vi "dataUnwrapperToplevel.vi"(0 "dataIn":u32[](array[numeric])=[814743552, 16777221, 16777621, 16778021, 814745600, 16777221, 16777621, 16778021, 814747648, 16777221, 16777621, 16778021, 814749696, 16777221, 16777621, 16778021, 814751744, 16777221, 16777621, 16778021, 814753792, 16777221, 16777621, 16778021, 0] format="%032b", 2 "nOfSteps":i32=6, 4 "nOfScans":i32=1) -> (10 "DataUntouchedOut":u32[](array[numeric]), 14 "VoltArray":u32[](array[numeric]) format="%032b", 16 "CounterArray":u32[][][](array[numeric]), 18 "TRSArray":u32[][][](array[numeric]))   [LabVIEW 2014]
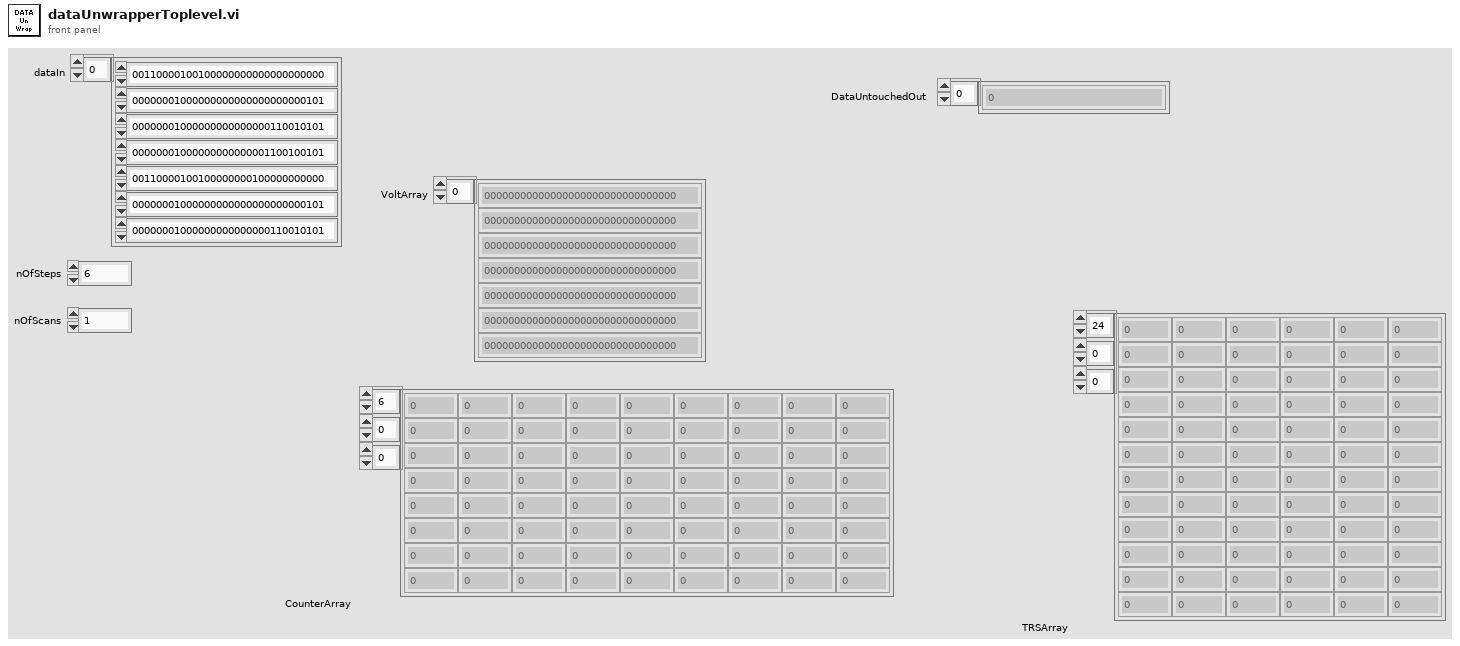
[diagram p1: front panel]
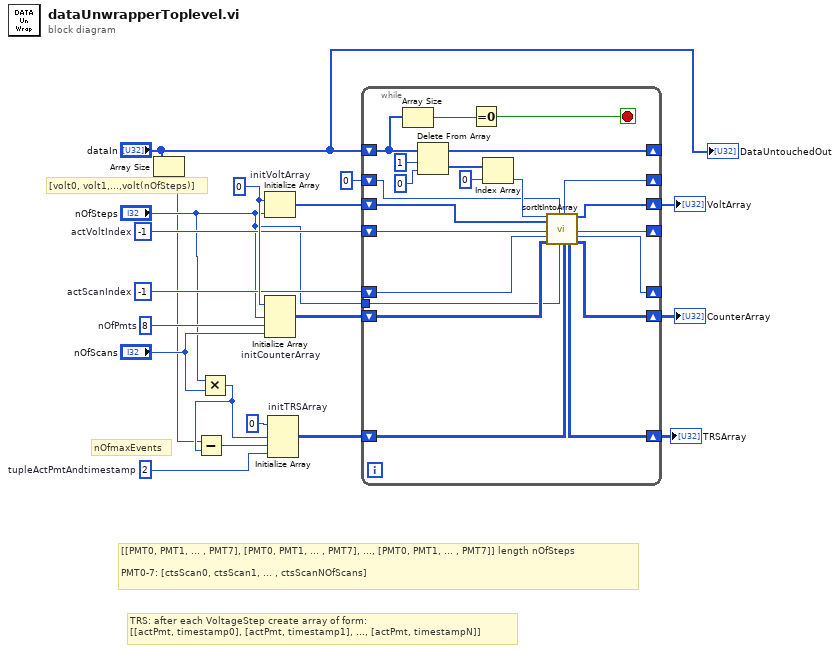
[diagram p0: block diagram]
diagram:
  w9 = 2  # tupleActPmtAndtimestamp
  w12 = -1  # actScanIndex
  w13 = -1  # actVoltIndex
  w19 = u32 0 ("element")
  w18 = 8  # nOfPmts
  # "nOfmaxEvents"
  # "TRS: after each VoltageStep create array of form:\n[[actPmt, timestamp0], [actPmt, timestamp1], ..., [actPmt, timestampN]]"
  # "[[PMT0, PMT1, ... , PMT7], [PMT0, PMT1, ... , PMT7], ..., [PMT0, PMT1, ... , PMT7]] length nOfSteps\n\nPMT0-7: [ctsScan0, ctsScan1, ... , ctsScanNOfScans]"
  # "[volt0, volt1,...,volt(nOfSteps)]"
  n1 = Array Size(array="dataIn") -> (size(s)=w2:i32)
  n2 = Multiply(x="nOfSteps", y="nOfScans") -> (x*y=w3:i32)
  n3 = Subtract(x=w2, y=w3) -> (x-y=w1:i32)
  n4 = Initialize Array "initVoltArray"(w19, "nOfSteps") -> (w16:u32[])
  n5 = Initialize Array "initCounterArray"(w19, "nOfSteps", w18, "nOfScans") -> (w17:u32[][][])
  n6 = Initialize Array "initTRSArray"(u32 0 ("element"), w3, w1, w9) -> (w10:u32[][][])
  n7 = while {
    shift-right: [w39] -> _
    shift-left: "dataIn" -> [w38]
    shift-right: [w27] -> w15
    shift-left: w16 -> [w32]
    shift-right: [w29] -> w14
    shift-left: w17 -> [w30]
    shift-right: [w28] -> _
    shift-left: w13 -> [w31]
    shift-right: [w25] -> _
    shift-left: w12 -> [w26]
    tunnel: "nOfSteps" -> [w24]
    shift-right: [w22] -> w6
    shift-left: w10 -> [w23]
    shift-right: [w21] -> _
    shift-left: 0 ("actEventIndexOut") -> [w20]
    stop <- w36 stop-if-true
    n8 = Array Size(array=w38) -> (size(s)=w37:i32)
    n9 = Delete From Array(array=w38, length=1, index=0) -> (deleted portion=w35:u32[], array with subset deleted=w39:u32[])
    n10 = Equal To 0?(x=w37) -> (x = 0?=w36:bool)
    n11 = Index Array(array=w35, index=0) -> (element=w33:u32)
    n12 = call "sortItIntoArray.vi"("element"=w33, "VoltArray"=w32, "actVoltIndex"=w31, "actScanIndex"=w26, "CounterArray"=w30, "actEventIndex"=w20, "nOfSteps"=w24, "TRSArrayIn"=w23) -> ("actEventIndexOut"=w21:i32, "TRSArrayOut"=w22:u32[][][], "VoltArrayOut"=w27:u32[], "actVoltIndexOut"=w28:i32, "actScanIndexOut"=w25:i32, "CounterArrayOut"=w29:u32[][][])  [unwired: 6 in]
  }
  "VoltArray" <- w15
  "CounterArray" <- w14
  "TRSArray" <- w6
  "DataUntouchedOut" <- "dataIn"
